vi "Parse Measurement Data.vi"(6 "Waveform Template":waveform(dbl), 8 "error in":errorcluster, 9 "Current":dbl[](array[numeric]), 10 "Voltage":dbl[](array[numeric]), 11 "PowerSupply in":refnum<class "PowerSupply.lvclass">) -> (0 "error out":errorcluster, 3 "PowerSupply out":refnum<class "PowerSupply.lvclass">)   [LabVIEW 2019, in "PowerSupply.lvlib" / "PowerSupply.lvclass"]
uses:
  Library/PowerSupply.lvclass
  C:/Users/Public/Documents/Development/builds/Instruments/Instruments.lvlibp/Library/Instruments.lvclass
  Library/PowerSupply.lvclass/PowerSupply.ctl
  Accessors/Read Status Flags.vi
  Accessors/Read Measured Table.vi
  Accessors/Write Measured Table.vi
  Accessors/Read Channel Names.vi
  builds/Instruments/Instruments.lvlibp/Accessors/Write Measured.vi
  builds/Instruments/Instruments.lvlibp/Library/Instruments.lvclass
panel:
  in  "Waveform Labels":T1(ring)
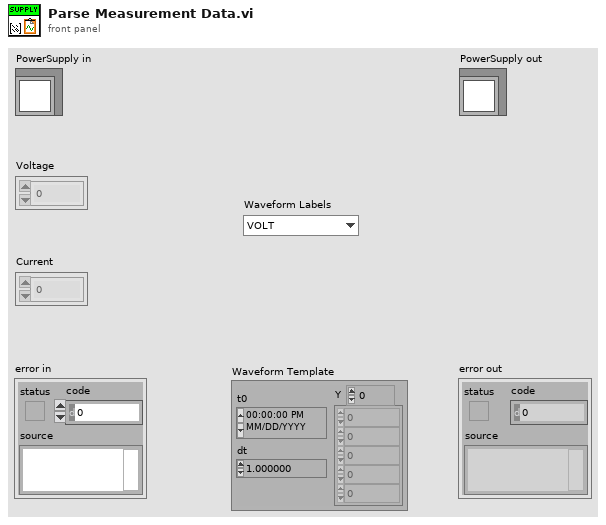
[diagram p1: front panel]
types:
  T1 = enum16{"VOLT", "AMP", "OUT", "OCP", "OVP", "INTLK"}
  T2 = typedef "PowerSupply.lvlibp/PowerSupply.lvclass/Status_Flags.ctl" = cluster{"Interlock":bool, "OVP":bool, "OCP":bool, "Output":bool}
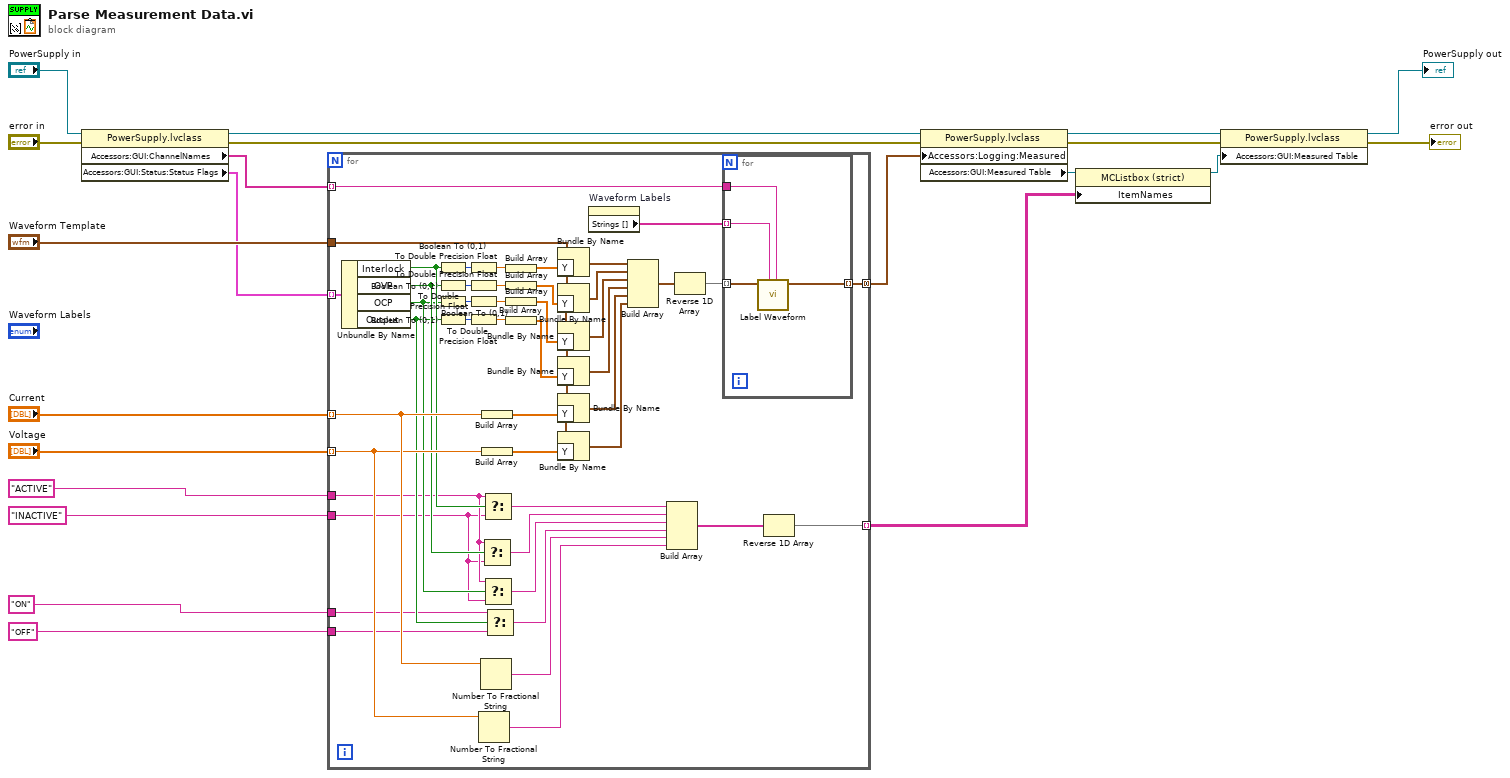
[diagram p0: block diagram]
diagram:
  n1 = property class="PowerSupply.lvclass"(reference="PowerSupply in", error in="error in") -> (reference out=w5:refnum<class "PowerSupply.lvclass">, error out=w10:errorcluster, "Accessors:GUI:ChannelNames"=w7:string[], "Accessors:GUI:Status:Status Flags"=w6:T2[])
  n2 = for {
    tunnel: "Voltage" -> [w47] mode=indexing
    tunnel: "Current" -> [w48] mode=indexing
    tunnel: w6 -> [w66] mode=indexing
    tunnel: w7 -> [w29] mode=indexing
    tunnel: "Waveform Template" -> [w60]
    tunnel: [w30] -> w9 mode=concatenating
    tunnel: "ACTIVE" -> [w42]
    tunnel: "ON" -> [w41]
    tunnel: "INACTIVE" -> [w40]
    tunnel: "OFF" -> [w39]
    tunnel: [w26] -> w19 mode=indexing
    n3 = Unbundle By Name(w66) -> ("Interlock"=w46:bool, "OVP"=w45:bool, "OCP"=w44:bool, "Output"=w43:bool)
    n4 = Boolean To (0,1)(Boolean=w46) -> (0, 1=w65:i16)
    n5 = Boolean To (0,1)(Boolean=w45) -> (0, 1=w64:i16)
    n6 = Boolean To (0,1)(Boolean=w44) -> (0, 1=w63:i16)
    n7 = Boolean To (0,1)(Boolean=w43) -> (0, 1=w62:i16)
    n8 = To Double Precision Float(number=w65) -> (double precision float=w25:dbl)
    n9 = To Double Precision Float(number=w64) -> (double precision float=w24:dbl)
    n10 = To Double Precision Float(number=w63) -> (double precision float=w23:dbl)
    n11 = To Double Precision Float(number=w62) -> (double precision float=w22:dbl)
    n12 = Number To Fractional String(number=w47) -> (F-format string=w33:string)  [unwired: 3 in]
    n13 = Number To Fractional String(number=w48) -> (F-format string=w34:string)  [unwired: 3 in]
    n14 = Build Array(w48) -> (w56:dbl[])
    n15 = Build Array(w47) -> (w55:dbl[])
    n16 = Select(t=w42, s=w45, f=w40) -> (s? t:f=w37:string)
    n17 = Select(t=w42, s=w46, f=w40) -> (s? t:f=w38:string)
    n18 = Select(t=w42, s=w44, f=w40) -> (s? t:f=w36:string)
    n19 = Select(t=w41, s=w43, f=w39) -> (s? t:f=w35:string)
    n20 = Build Array(w25) -> (w61:dbl[])
    n21 = Build Array(w24) -> (w59:dbl[])
    n22 = Build Array(w23) -> (w58:dbl[])
    n23 = Build Array(w22) -> (w57:dbl[])
    n24 = Bundle By Name(cluster=w60, "Y"=w61) -> (w54:waveform(dbl))
    n25 = Bundle By Name(cluster=w60, "Y"=w59) -> (w53:waveform(dbl))
    n26 = Bundle By Name(cluster=w60, "Y"=w58) -> (w52:waveform(dbl))
    n27 = Bundle By Name(cluster=w60, "Y"=w57) -> (w51:waveform(dbl))
    n28 = Bundle By Name(cluster=w60, "Y"=w56) -> (w50:waveform(dbl))
    n29 = Bundle By Name(cluster=w60, "Y"=w55) -> (w49:waveform(dbl))
    n30 = property on="Waveform Labels" class="Enum (strict)"() -> ("Strings []"=w27:string[])  [unwired: 2 in, 2 out]
    n31 = Build Array(w54, w53, w52, w51, w50, w49) -> (w31:waveform(dbl)[])
    n32 = Build Array(w38, w37, w36, w35, w34, w33) -> (w32:string[])
    n33 = Reverse 1D Array(array=w31) -> (reversed array=w28:waveform(dbl)[])
    n34 = for {
      tunnel: w28 -> [w70] mode=indexing
      tunnel: [w69] -> w30 mode=indexing
      tunnel: w29 -> [w68]
      tunnel: w27 -> [w67] mode=indexing
      n35 = call "Label Waveform.vi"("Unique Channel Name"=w68, "Measurement"=w67, "Input waveform"=w70) -> ("Labelled Waveform"=w69:waveform(dbl))  [unwired: 8 in]
    }
    n36 = Reverse 1D Array(array=w32) -> (reversed array=w26:string[])
  }
  n37 = property class="PowerSupply.lvclass"(reference=w5, error in=w10, "Accessors:Logging:Measured"=w9) -> (reference out=w16:refnum<class "PowerSupply.lvclass">, error out=w15:errorcluster, "Accessors:GUI:Measured Table"=w17:refnum<vi>)
  n38 = property class="MCListbox (strict)"(reference=w17, "ItemNames"=w19) -> (reference out=w18:refnum<vi>)  [unwired: 1 in, 1 out]
  n39 = property class="PowerSupply.lvclass"(reference=w16, error in=w15, "Accessors:GUI:Measured Table"=w18) -> (reference out=→"PowerSupply out":refnum<class "PowerSupply.lvclass">, error out=→"error out":errorcluster)
